vi "maxTrigVel.vi"(1 "stepSize (mm)":dbl) -> (0 "maxVel (mm/s)":dbl)   [LabVIEW 2015]
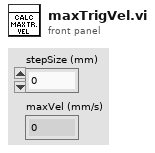
[diagram p1: front panel]
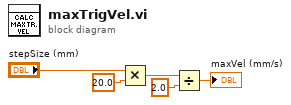
[diagram p0: block diagram]
diagram:
  n1 = Multiply(x="stepSize (mm)", y=20.0) -> (x*y=w3:dbl)
  n2 = Divide(x=w3, y=2.0) -> (x/y=→"maxVel (mm/s)":dbl)
